vi "Mean Replace.vi"() -> ()   [LabVIEW 2020]
panel:
  out "结果字符串":string
  in  "Formular":string
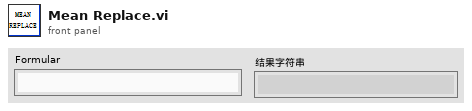
[diagram p1: front panel]
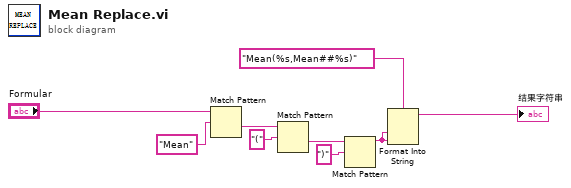
[diagram p0: block diagram]
diagram:
  n1 = Match Pattern(string="Formular", regular expression="Mean" ("正则表达式")) -> (after substring=w7:string)  [unwired: 1 in, 3 out]
  n2 = Match Pattern(string=w7, regular expression="(" ("正则表达式")) -> (after substring=w4:string)  [unwired: 1 in, 3 out]
  n3 = Match Pattern(string=w4, regular expression=")" ("正则表达式")) -> (before substring=w2:string)  [unwired: 1 in, 3 out]
  n4 = Format Into String(format string="Mean(%s,Mean##%s)" ("格式字符串"), w2, w2) -> (resulting string=→"结果字符串":string)  [unwired: 2 in, 1 out]
